vi "K_S30_VISA CloseComPort.vi"(4 "error in (not connected)":errorcluster caption="Fehler (Eingang - kein Fehler)") -> (0 "Fehlerausgang":errorcluster)   [LabVIEW 2013]
uses:
  K_S30_VISA Global.vi
panel:
  # "Close the serial Port\nV1.0, b.v."
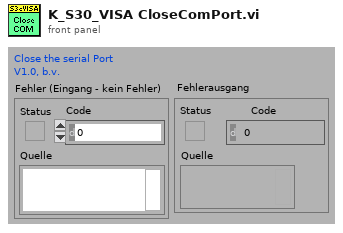
[diagram p1: front panel]
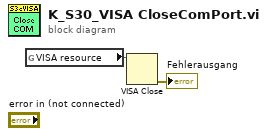
[diagram p0: block diagram]
diagram:
  n1 = global read "K_S30_VISA Global.vi" "VISA resource"() -> (w1:refnum<visa-resource-name>)
  n2 = VISA Close(VISA resource name=w1) -> (error out=→"Fehlerausgang":errorcluster)  [unwired: 1 in]
